vi "to string.vi"(8 "error in":errorcluster, 11 "fixed channel configuration in":refnum<class "BuckBoost configuration.lvclass">) -> (0 "error out":errorcluster, 1 "data":string, 2 "version":string, 3 "fixed channel configuration out":refnum<class "BuckBoost configuration.lvclass">)   [LabVIEW 2017, in "BuckBoost configuration.lvclass"]
doc: "Provides an interface for saving a module configuration to a file or other serialized data source. It is recommended that all children of this class store data in two sets--data required for its own initialization, and any data required for parent initialization--and that each implementation uses the <b>Call Parent Method</b> primitive to serialize parent information.\nNI Tag Bus Module Framework 1.0.3.43\nNI Systems Engineering"
uses:
  BuckBoost configuration.lvclass
  BuckBoost configuration.lvclass/BuckBoost configuration.ctl
  <vilib>/NI/JSON Support for LabVIEW/JSON Data Classes/JSON Object/New JSON Object (Empty).vi
  <vilib>/NI/JSON Support for LabVIEW/JSON Data Classes/JSON Object/Insert Key Value Pair (Single).vi
  <vilib>/NI/DCAF/Tag Editor Core/control module/configuration/control module configuration.lvclass
  <vilib>/NI/JSON Support for LabVIEW/JSON Data Classes/JSON Object/JSON Object.lvclass
  <vilib>/NI/JSON Support for LabVIEW/JSON Data Classes/JSON Helper/JSON Helper.lvclass
  <vilib>/NI/Configuration Framework/serializable configuration/NISE_CEF_serializable configuration.lvclass
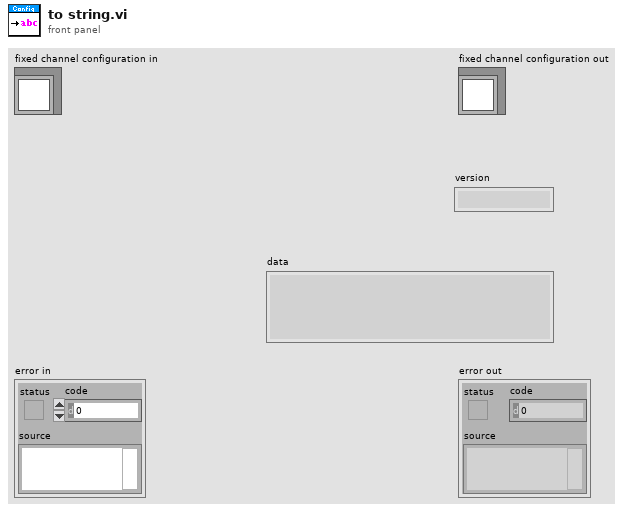
[diagram p1: front panel]
types:
  T1 = typedef "BuckBoostInterface.lvlib/TuningParameters.ctl" = cluster{"gains":T2, "manualInput":sgl, "rampRate":sgl, "pertAmp":sgl, "pertFreq":sgl, "controlFreq":sgl, "state":T3}
  T2 = typedef "niFpgaPID_PIGains.ctl" = cluster{"proportional gain":sgl, "integral gain":sgl}
  T3 = typedef "BuckBoost.lvlib/contState.ctl" = enum16{"disabled", "manual", "normal", "perturb"}
  T4 = typedef "BuckBoostInterface.lvlib/modulationConfig.ctl" = cluster{"SwitchingSpeed":dbl, "Deadband":dbl, "modulationRate":dbl}
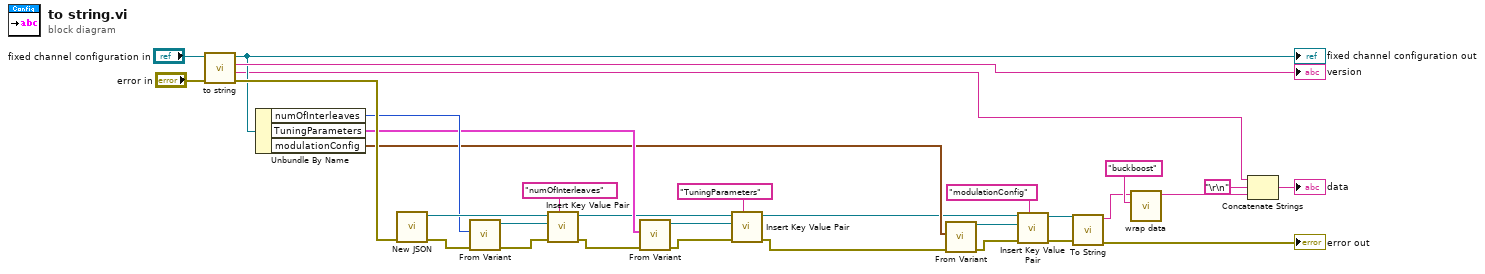
[diagram p0: block diagram]
diagram:
  n1 = call-parent "to string.vi"("error in"="error in", "fixed channel configuration in"="fixed channel configuration in") -> ("error out"=w29:errorcluster, "data"=w7:string, "version"=→"version":string, "fixed channel configuration out"=w28:refnum<class "BuckBoost configuration.lvclass">)  [unwired: 6 in]
  "fixed channel configuration out" <- w28
  n2 = Unbundle By Name(w28) -> ("numOfInterleaves"=w24:u8, "TuningParameters"=w20:T1, "modulationConfig"=w15:T4)
  n3 = call-poly <vilib>:"New JSON.vi"("error in (no error)"=w29) -> ("error out"=w23:errorcluster, "JSON Object out"=w25:refnum<class "JSON Object.lvclass">)  [unwired: 9 in]
  n4 = call <vilib>:"From Variant.vi"("error in (no error)"=w23, "Variant"=w24) -> ("error out"=w22:errorcluster, "JSON out"=w21:refnum<class "JSON Null.lvclass">)  [unwired: 8 in]
  n5 = call-poly <vilib>:"Insert Key Value Pair.vi"("key"="numOfInterleaves", "error in (no error)"=w22, "value"=w21, "JSON Object in"=w25) -> ("error out"=w18:errorcluster, "JSON Object out"=w19:refnum<class "JSON Object.lvclass">)  [unwired: 5 in, 1 out]
  n6 = call <vilib>:"From Variant.vi"("error in (no error)"=w18, "Variant"=w20) -> ("error out"=w16:errorcluster, "JSON out"=w17:refnum<class "JSON Null.lvclass">)  [unwired: 8 in]
  n7 = call-poly <vilib>:"Insert Key Value Pair.vi"("key"="TuningParameters", "error in (no error)"=w16, "value"=w17, "JSON Object in"=w19) -> ("error out"=w1:errorcluster, "JSON Object out"=w2:refnum<class "JSON Object.lvclass">)  [unwired: 5 in, 1 out]
  n8 = call <vilib>:"From Variant.vi"("error in (no error)"=w1, "Variant"=w15) -> ("error out"=w14:errorcluster, "JSON out"=w13:refnum<class "JSON Null.lvclass">)  [unwired: 8 in]
  n9 = call-poly <vilib>:"Insert Key Value Pair.vi"("key"="modulationConfig", "error in (no error)"=w14, "value"=w13, "JSON Object in"=w2) -> ("error out"=w11:errorcluster, "JSON Object out"=w10:refnum<class "JSON Object.lvclass">)  [unwired: 5 in, 1 out]
  n10 = call-dynamic "To String.vi"("error in (no error)"=w11, "JSON Object in"=w10) -> ("error out"=→"error out":errorcluster, "String"=w5:string)  [unwired: 8 in]
  n11 = call <vilib>:"wrap data.vi"("identifier"="buckboost", "data to wrap"=w5) -> ("wrapped data"=w8:string)  [unwired: 9 in]
  n12 = Concatenate Strings(w7, "\r\n", w8) -> (→"data":string)
